vi "BRig_RT_comm_webdav_upload__buildPath.vi"(9 "input_fileName_prefix":string, 10 "input_fileName":string="dataTrial") -> (0 "output_localPath":path, 1 "output_targetPath_spare":string, 2 "output_targetPath":string)   [LabVIEW 2014]
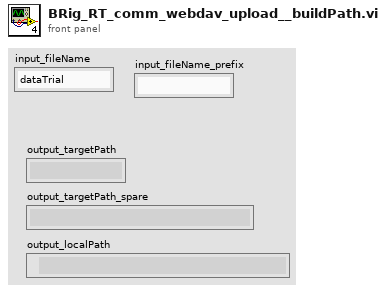
[diagram p1: front panel]
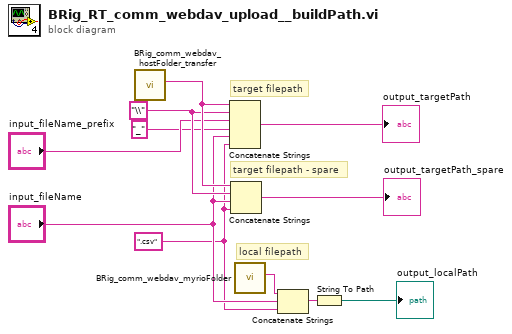
[diagram p0: block diagram]
diagram:
  w8 = "\\" ("string")
  w4 = ".csv" ("string")
  # "target filepath"
  # "target filepath - spare"
  # "local filepath"
  n1 = call "BRig_comm_webdav_hostFolder_transfer.vi"() -> ("output_HostFolder"=w9:string)  [unwired: 11 in]
  n2 = Concatenate Strings(w9, w8, "input_fileName_prefix", "_" ("string"), "input_fileName", w4) -> (→"output_targetPath":string)
  n3 = Concatenate Strings(w9, w8, "input_fileName", w4) -> (→"output_targetPath_spare":string)
  n4 = call "BRig_comm_webdav_myrioFolder.vi"() -> ("output_myrioFolder"=w10:string)  [unwired: 11 in]
  n5 = Concatenate Strings(w10, "input_fileName", w4) -> (w11:string)
  n6 = String To Path(string=w11) -> (path=→"output_localPath":path)
